vi "Add Items to ListView by Text and ImageIndex Array.vi"(8 "error in (no error)":errorcluster caption="错误输入（无错误）", 9 "ImageIndex":i32[](array[numeric]), 10 "Text":string[](array[string]), 11 "ListViewClass 输入":refnum<class "ListViewClass.lvclass"> caption="DNL_LabVIEW Object in") -> (0 "error out":errorcluster caption="错误输出", 3 "ListViewClass 输出":refnum<class "ListViewClass.lvclass"> caption="DNL_LabVIEW Object out")   [LabVIEW 2012, in "ListViewClass.lvclass"]
uses:
  ListViewClass.lvclass
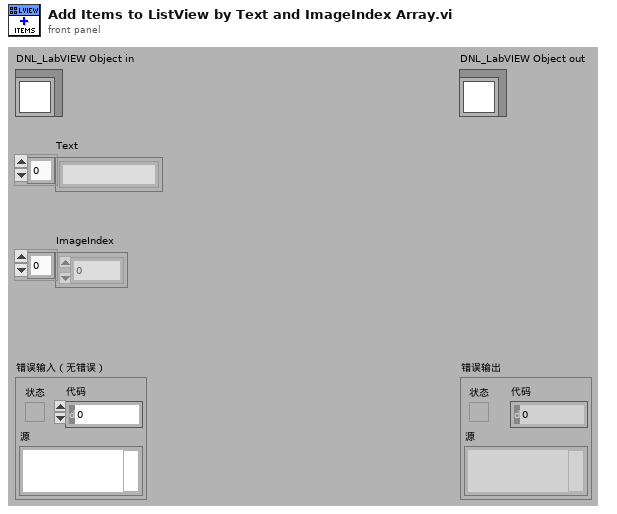
[diagram p1: front panel]
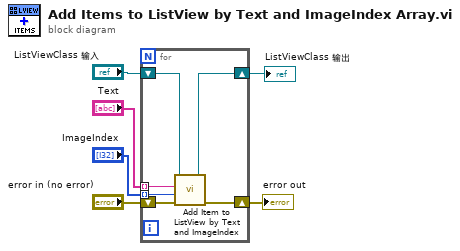
[diagram p0: block diagram]
diagram:
  n1 = for {
    shift-right: [w11] -> w5
    shift-left: "ListViewClass 输入" -> [w12]
    shift-right: [w9] -> w3
    shift-left: "error in (no error)" -> [w10]
    tunnel: "Text" -> [w8] mode=indexing
    tunnel: "ImageIndex" -> [w7] mode=indexing
    n2 = call "Add Item to ListView by Text and ImageIndex.vi"("error in (no error)"=w10, "imageIndex"=w7, "text"=w8, "ListViewClass 输入"=w12) -> ("error out"=w9:errorcluster, "ListViewClass 输出"=w11:refnum<class "ListViewClass.lvclass">)  [unwired: 6 in]
  }
  "error out" <- w3
  "ListViewClass 输出" <- w5
